vi "CAD@MotionTable2Points__Parameter.vi"(1 "ParamterIn":string) -> (0 "ParamterOut":string)   [LabVIEW 2020]
panel:
  in  "WorkingSpace":string(combo)
  in  "Simulate":string(combo)
  in  "Point":string(combo)
  in  "Robot":string(combo)
  in  "Confirm":bool
  # "CAD@MotionTable2Points $Robot,$Point,$Simulate(,$WorkingSpace)"
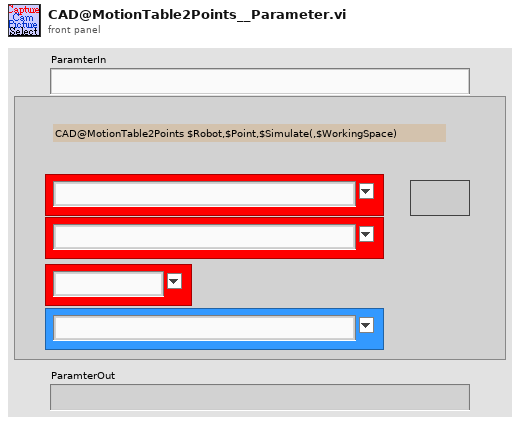
[diagram p1: front panel]
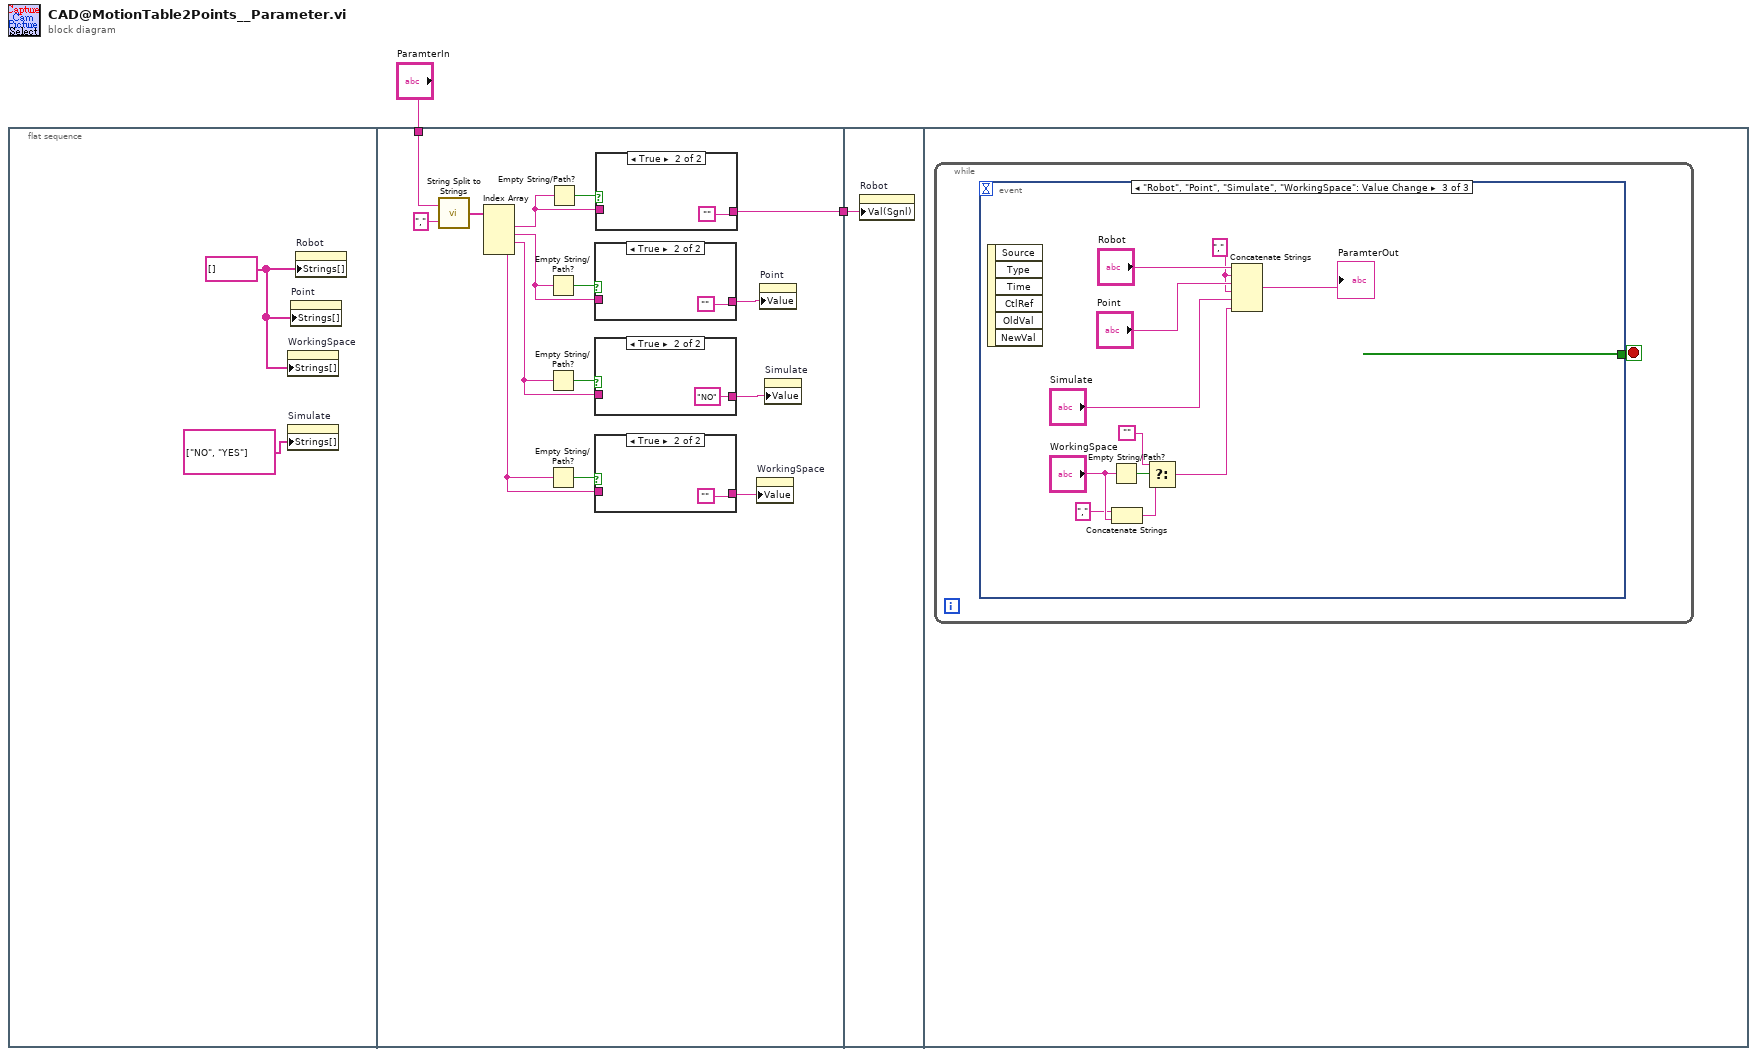
[diagram p0: block diagram]
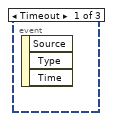
[diagram p6: hidden frame]
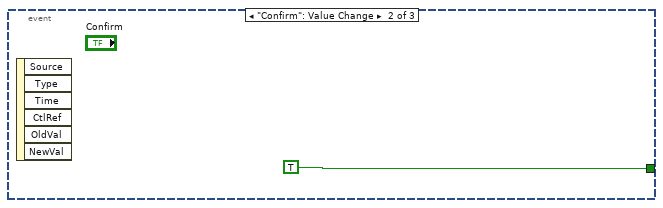
[diagram p7: hidden frame]
diagram:
  n1 = flat-sequence {
    tunnel: "ParamterIn" -> [w17]
    tunnel: [w18] -> w1
    tunnel: w1 -> [w28]
    frame #0 {
      w3 = string[] [] ("Strings []")
      n2 = property on="WorkingSpace" class="CmbBox"("Strings[]"=w3) -> ()  [unwired: 2 in, 2 out]
      n3 = property on="Simulate" class="CmbBox"("Strings[]"=string[] ["NO", "YES"] ("Strings []")) -> ()  [unwired: 2 in, 2 out]
      n4 = property on="Point" class="CmbBox"("Strings[]"=w3) -> ()  [unwired: 2 in, 2 out]
      n5 = property on="Robot" class="CmbBox"("Strings[]"=w3) -> ()  [unwired: 2 in, 2 out]
    }
    frame #1 {
      n6 = call "String Split to Strings.vi"("search string/char (-)"=",", "String"=w17) -> ("Array"=w15:string[])
      n7 = Index Array(array=w15) -> (element #1=w14:string, element #2=w12:string, element #3=w8:string, element #4=w6:string)  [unwired: 4 in]
      n8 = Empty String/Path?(string/path=w12) -> (empty?=w13:bool)
      n9 = Empty String/Path?(string/path=w8) -> (empty?=w10:bool)
      n10 = Empty String/Path?(string/path=w6) -> (empty?=w7:bool)
      n11 = Empty String/Path?(string/path=w14) -> (empty?=w19:bool)
      n12 = case shown="True" w13 {
        tunnel: w12 -> [w24 _]
        tunnel: [w24 ""] -> w11
        frame False {
        }
        frame True {
        }
      }
      n13 = case shown="True" w10 {
        tunnel: w8 -> [w22 _]
        tunnel: [w22 "NO"] -> w9
        frame False {
        }
        frame True {
        }
      }
      n14 = case shown="True" w7 {
        tunnel: w6 -> [w20 _]
        tunnel: [w20 ""] -> w5
        frame False {
        }
        frame True {
        }
      }
      n15 = case shown="True" w19 {
        tunnel: w14 -> [w26 _]
        tunnel: [w26 ""] -> w18
        frame False {
        }
        frame True {
        }
      }
      n16 = property on="WorkingSpace" class="CmbBox"("Value"=w5) -> ()  [unwired: 2 in, 2 out]
      n17 = property on="Point" class="CmbBox"("Value"=w11) -> ()  [unwired: 2 in, 2 out]
      n18 = property on="Simulate" class="CmbBox"("Value"=w9) -> ()  [unwired: 2 in, 2 out]
    }
    frame #2 {
      n19 = property on="Robot" class="CmbBox"("Val(Sgnl)"=w28) -> ()  [unwired: 2 in, 2 out]
    }
    frame #3 {
      n20 = while {
        stop <- w29 stop-if-true
        n21 = event shown="[2] \"Robot\", \"Point\", \"Simulate\", \"WorkingSpace\": Value Change" {
          selector: _ -> [_ _ _]
          dyn-events: _ -> [_ _ _]
          timeout: _ -> [_ _ _]
          tunnel: [_ TRUE _] -> w29
          event Timeout {
            n22 = event-data() -> ()  [unwired: 1 in, 3 out]
          }
          event "Confirm": Value Change {
            n23 = event-data() -> ()  [unwired: 1 in, 6 out]
          }
          event "Robot", "Point", "Simulate", "WorkingSpace": Value Change {
            w38 = ","
            n24 = event-data() -> ()  [unwired: 1 in, 6 out]
            n25 = Empty String/Path?(string/path="WorkingSpace") -> (empty?=w36:bool)
            n26 = Concatenate Strings("," ("string"), "WorkingSpace") -> (w33:string)
            n27 = Select(t="", s=w36, f=w33) -> (s? t:f=w31:string)
            n28 = Concatenate Strings("Robot", w38, "Point", w38, "Simulate", w31) -> (→"ParamterOut":string)
          }
        }
      }
    }
  }
